vi "Get All Controls Recursively.vi"(5 "Owner Labels":string[](array[string]), 7 "Owner Classes":string[](array[string]), 8 "error in (no error)":errorcluster, 9 "Subpanel?":bool, 10 "Control Map":map{string, T1[]}(c390), 11 "VI Ref":refnum<vi>) -> (0 "error out":errorcluster, 2 "Control Map out":map{string, T1[]}(c390), 3 "VI Ref out":refnum<vi>)   [LabVIEW 2020, in "MacroAssert.lvlib"]
doc: "Gets all control references within <B>VI Ref</B> recursively by checking it for subpanels, getting any controls in them, checking for nested subpanels, etc."
uses:
  MacroAssert.lvlib
  CTLs/Control Map Control Data.ctl
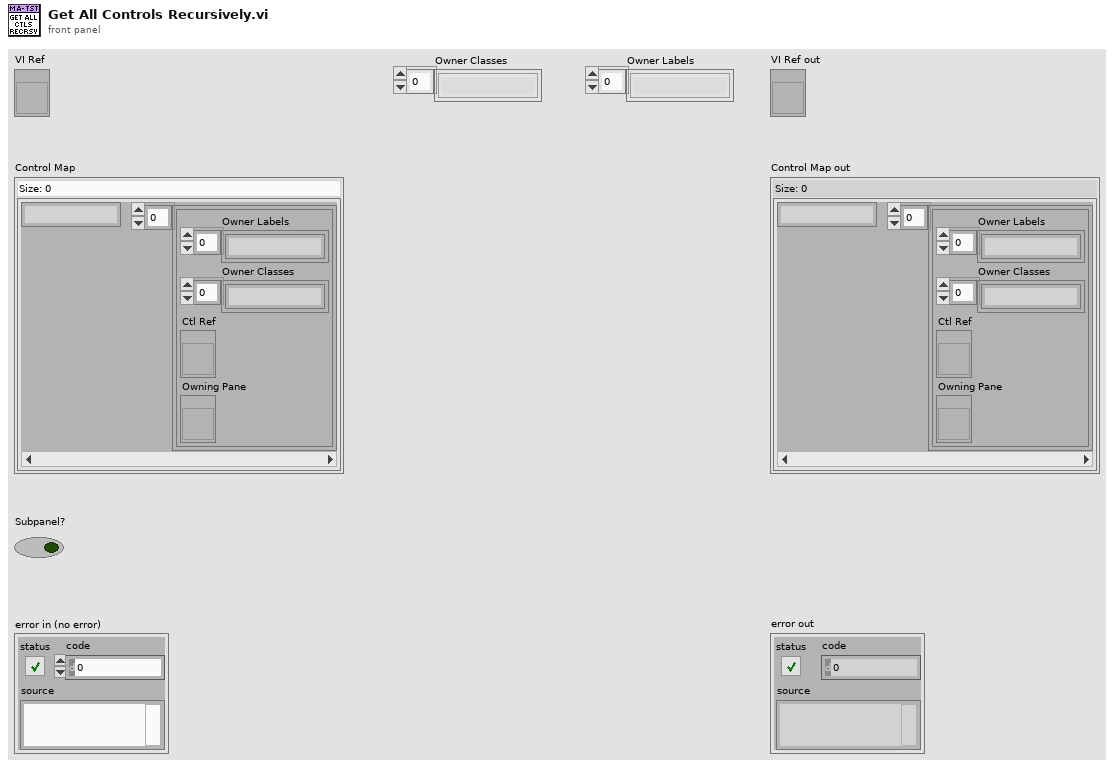
[diagram p1: front panel]
types:
  T1 = typedef "MacroAssert.lvlib/Control Map Control Data.ctl" = cluster{"Owner Labels":string[], "Owner Classes":string[], "Ctl Ref":refnum<vi>, "Owning Pane":refnum<vi>}
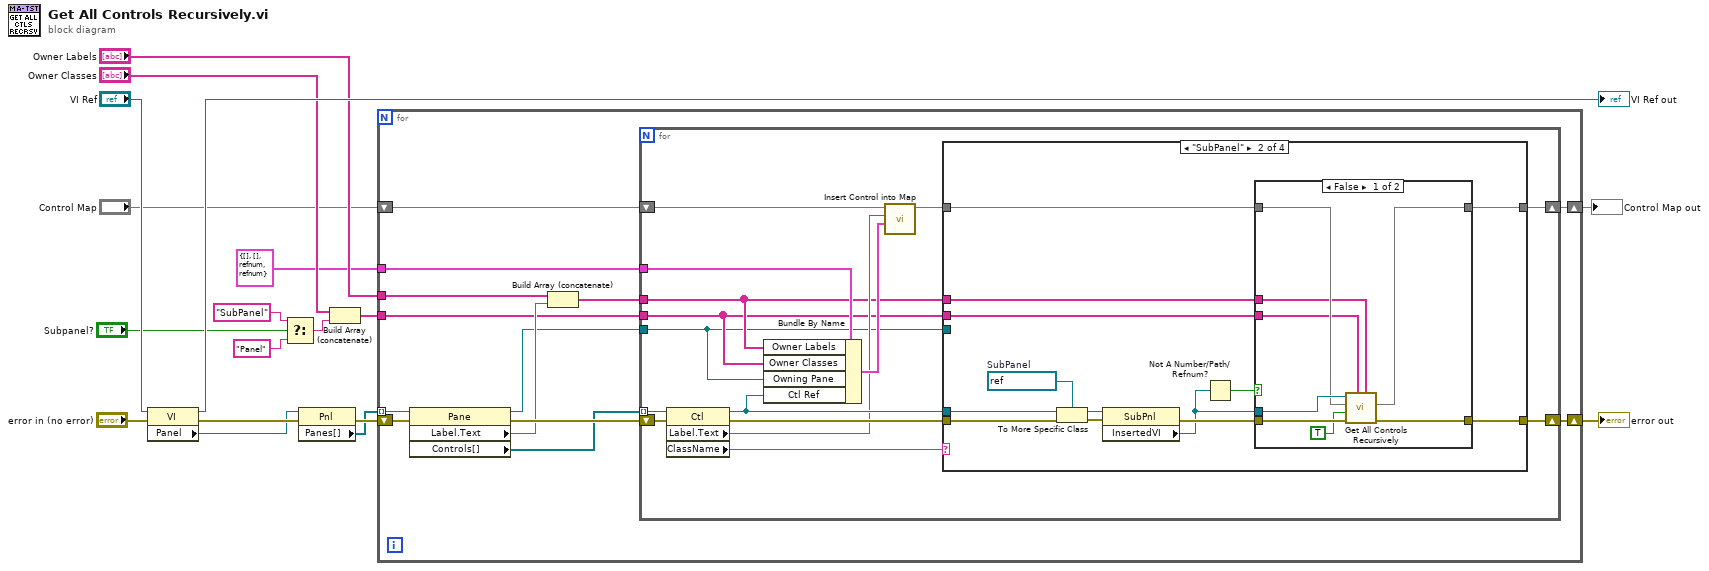
[diagram p0: block diagram]
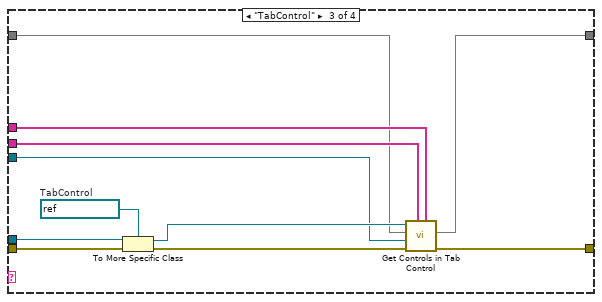
[diagram p4: hidden frame]
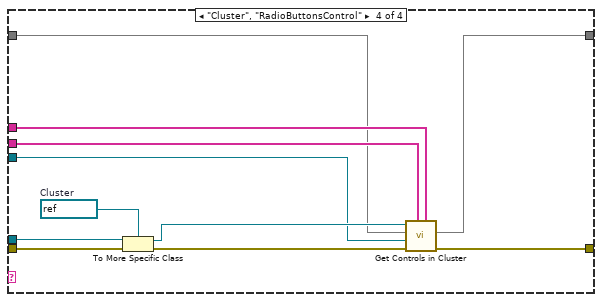
[diagram p5: hidden frame]
diagram:
  n1 = property class="VI"(reference="VI Ref", error in="error in (no error)") -> (reference out=→"VI Ref out":refnum<vi>, error out=w18:errorcluster, "Panel"=w12:refnum<vi>)
  n2 = Select(t="SubPanel", s="Subpanel?", f="Panel") -> (s? t:f=w1:string)
  n3 = property class="Pnl"(reference=w12, error in=w18) -> (error out=w13:errorcluster, "Panes[]"=w11:refnum<vi>[])  [unwired: 1 out]
  n4 = Build Array (concatenate)("Owner Classes", w1) -> (w9:string[])
  n5 = for {
    tunnel: w11 -> [w29] mode=indexing
    shift-right: [w28] -> w15
    shift-left: w13 -> [w31]
    tunnel: w9 -> [w24]
    tunnel: "Owner Labels" -> [w27]
    tunnel: T1 {"Owner Labels"=[], "Owner Classes"=[], "Ctl Ref"=refnum, "Owning Pane"=refnum} ("Ctl Data") -> [w21]
    shift-right: [w20] -> w5
    shift-left: "Control Map" -> [w22]
    n6 = property class="Pane"(reference=w29, error in=w31) -> (reference out=w19:refnum<vi>, error out=w30:errorcluster, "Label.Text"=w26:string, "Controls[]"=w23:refnum<vi>[])
    n7 = Build Array (concatenate)(w27, w26) -> (w25:string[])
    n8 = for {
      shift-right: [w46] -> w28
      shift-left: w30 -> [w44]
      tunnel: w23 -> [w45] mode=indexing
      tunnel: w25 -> [w34]
      tunnel: w24 -> [w33]
      tunnel: w21 -> [w35]
      shift-right: [w42] -> w20
      shift-left: w22 -> [w40]
      tunnel: w19 -> [w32]
      n9 = property class="Ctl"(reference=w45, error in=w44) -> (reference out=w38:refnum<vi>, error out=w43:errorcluster, "Label.Text"=w37:string, "ClassName"=w36:string)
      n10 = Bundle By Name(cluster=w35, "Owner Labels"=w34, "Owner Classes"=w33, "Owning Pane"=w32, "Ctl Ref"=w38) -> (w41:T1)
      n11 = call "Insert Control into Map.vi"("Ctl Data"=w41, "Name"=w37, "Control Map"=w40) -> ("Control Map out"=w39:map{string, T1[]})  [unwired: 8 in]
      n12 = case shown="\"SubPanel\"" w36 {
        tunnel: [w48 w55 w78 w89] -> w46
        tunnel: w38 -> [_ w59 w81 w92]
        tunnel: w43 -> [w48 w58 w80 w91]
        tunnel: w39 -> [w47 w50 w74 w83]
        tunnel: [w47 w49 w73 w86] -> w42
        tunnel: w34 -> [_ w52 w75 w84]
        tunnel: w33 -> [_ w51 w76 w87]
        tunnel: w32 -> [_ _ w72 w85]
        frame Default {
        }
        frame "SubPanel" {
          w60 = refnum<vi> refnum  # SubPanel
          n13 = To More Specific Class(target class=w60, reference=w59, error in=w58) -> (specific class reference=w61:refnum<vi>, error out=w57:errorcluster)
          n14 = property class="SubPnl"(reference=w61, error in=w57) -> (error out=w56:errorcluster, "InsertedVI"=w53:refnum<vi>)  [unwired: 1 out]
          n15 = Not A Number/Path/Refnum?(number/path/refnum=w53) -> (NaN/Path/Refnum?=w54:bool)
          n16 = case shown="False" w54 {
            tunnel: w56 -> [w69 w71]
            tunnel: [w68 w71] -> w55
            tunnel: [w66 w70] -> w49
            tunnel: w53 -> [w67 _]
            tunnel: w52 -> [w64 _]
            tunnel: w51 -> [w63 _]
            tunnel: w50 -> [w65 w70]
            frame False {
              n17 = call "Get All Controls Recursively.vi"("Owner Labels"=w64, "Owner Classes"=w63, "error in (no error)"=w69, "Subpanel?"=TRUE, "Control Map"=w65, "VI Ref"=w67) -> ("error out"=w68:errorcluster, "Control Map out"=w66:map{string, T1[]})  [unwired: 3 in, 1 out]
            }
            frame True {
            }
          }
        }
        frame "TabControl" {
          w82 = refnum<vi> refnum  # TabControl
          n18 = To More Specific Class(target class=w82, reference=w81, error in=w80) -> (specific class reference=w77:refnum<vi>, error out=w79:errorcluster)
          n19 = call "Get Controls in Tab Control.vi"("Owner Labels"=w75, "Owner Classes"=w76, "error in (no error)"=w79, "Owning Pane"=w72, "Control Map"=w74, "TabCtl Ref"=w77) -> ("error out"=w78:errorcluster, "Control Map out"=w73:map{string, T1[]})  [unwired: 3 in, 1 out]
        }
        frame "Cluster", "RadioButtonsControl" {
          w93 = refnum<vi> refnum  # Cluster
          n20 = To More Specific Class(target class=w93, reference=w92, error in=w91) -> (specific class reference=w88:refnum<vi>, error out=w90:errorcluster)
          n21 = call "Get Controls in Cluster.vi"("Owner Labels"=w84, "Owner Classes"=w87, "error in (no error)"=w90, "Owning Pane"=w85, "Control Map"=w83, "Cluster Ref"=w88) -> ("error out"=w89:errorcluster, "Control Map out"=w86:map{string, T1[]})  [unwired: 3 in, 1 out]
        }
      }
    }
  }
  "error out" <- w15
  "Control Map out" <- w5
